vi "Create sel_energy Queues.vi"(8 "error in (no error)":errorcluster) -> (0 "error out":errorcluster, 3 "Message Queue":cluster{"Main":refnum<queue>})   [LabVIEW 2020, in "Front Panel Message Queue.lvlib"]
doc: "This VI creates and initializes all the message queues for your application. If your application requires more than one message queue, right-click the \"Message Queues\" constant above and select Open Type Def. Add the new Message Queue(s) to the type definition, then initialize them in this VI."
uses:
  Front Panel Message Queue.lvlib
  Message Cluster.ctl
  Enqueue Message (Single).vi
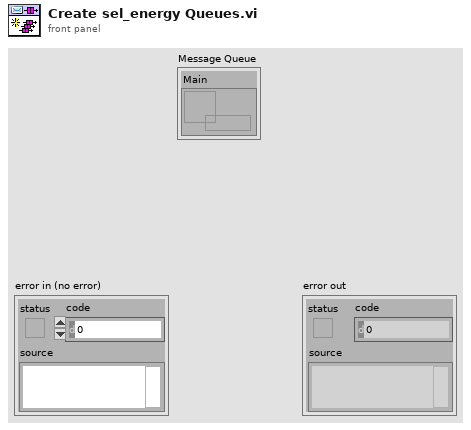
[diagram p1: front panel]
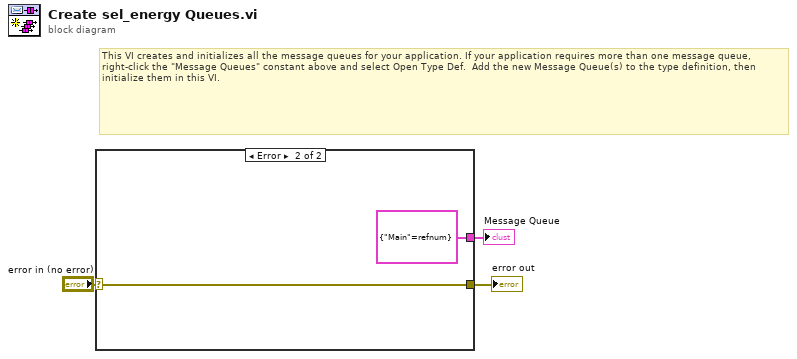
[diagram p0: block diagram]
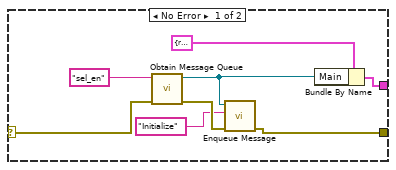
[diagram p2: hidden frame]
diagram:
  # "This VI creates and initializes all the message queues for your application. If your application requires more than one message queue, right-click the \"Message Queues\" constant above and select Open Type Def.  Add the new Message Queue(s) to the type definition, then initialize them in this VI."
  n1 = case shown="Error" "error in (no error)" {
    selector: "error in (no error)" -> [w7 w13]
    tunnel: [w8 w13] -> w3
    tunnel: [w11 cluster{"Main":refnum<queue>} {"Main"=refnum}] -> w1
    frame No Error {
      n2 = call "Obtain Message Queue.vi"("error in (no error)"=w7, "name"="sel_en") -> ("error out"=w10:errorcluster, "Message Queue"=w9:refnum<queue>)  [unwired: 8 in]
      n3 = call-poly "Enqueue Message.vi"("error in (no error)"=w10, "Message"="Initialize", "Message Queue"=w9) -> ("error out"=w8:errorcluster)  [unwired: 7 in, 1 out]
      n4 = Bundle By Name(cluster=cluster{"Main":refnum<queue>} {"Main"=refnum}, "Main"=w9) -> (w11:cluster{"Main":refnum<queue>})
    }
    frame Error {
    }
  }
  "error out" <- w3
  "Message Queue" <- w1
